vi "CalculateTorqueRipplevi.vi"(8 "error in (no error)":errorcluster, 11 "Torque Waveform":waveform(dbl)) -> (0 "error out":errorcluster, 3 "Torque Ripple (%)":dbl)   [LabVIEW 2017, in "McsaAnalysisFunctions.lvlib"]
uses:
  <vilib>/addons/InsightCM/Utilities/Analysis/MCSA/McsaAnalysisFunctions.lvlib
  <vilib>/Analysis/baseanly.llb/Mean (DBL).vi
  <vilib>/Waveform/WDTOps.llb/WDT Waveform Duration DBL.vi
  <vilib>/Waveform/WDTOps.llb/WDT Get Waveform Subset DBL.vi
  <vilib>/Analysis/NI_AALBase.lvlib
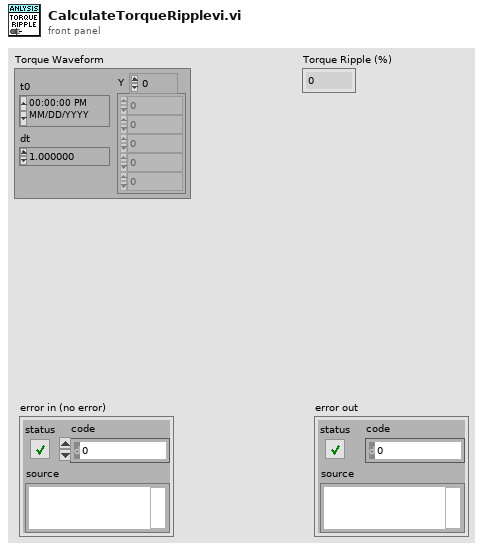
[diagram p1: front panel]
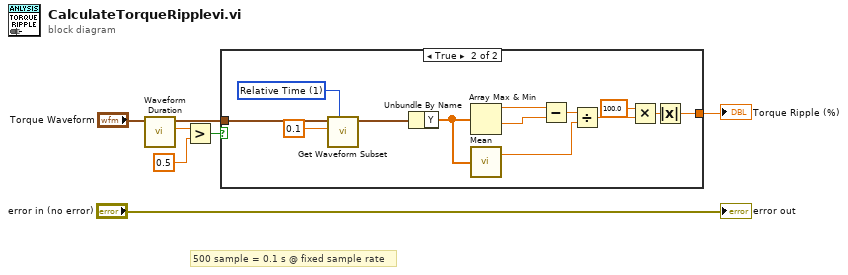
[diagram p0: block diagram]
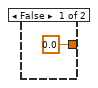
[diagram p2: hidden frame]
diagram:
  # "500 sample = 0.1 s @ fixed sample rate"
  n1 = call-poly <vilib>:"Waveform Duration.vi"("waveform in"="Torque Waveform") -> ("duration"=w5:dbl, "waveform out"=w6:waveform(dbl))  [unwired: 8 in, 1 out]
  n2 = Greater?(x=w5, y=0.5) -> (0:w2:bool)
  n3 = case shown="True" w2 {
    tunnel: w6 -> [_ w12]
    tunnel: [0.0 w11] -> w3
    frame False {
    }
    frame True {
      w10 = u16 1 items=["Samples", "Relative Time"] ("start/duration format")
      n4 = call-poly <vilib>:"Get Waveform Subset.vi"("start/duration format"=w10, "start samples/time"=0.1, "waveform in"=w12) -> ("waveform out"=w21:waveform(dbl))  [unwired: 3 in, 3 out]
      n5 = Unbundle By Name(w21) -> ("Y"=w20:dbl[])
      n6 = Array Max & Min(array=w20) -> (max value=w19:dbl, min value=w18:dbl)  [unwired: 2 out]
      n7 = call-poly <vilib>:"Mean.vi"("X"=w20) -> ("mean"=w16:dbl)  [unwired: 1 out]
      n8 = Subtract(x=w19, y=w18) -> (x-y=w17:dbl)
      n9 = Divide(x=w17, y=w16) -> (x/y=w15:dbl)
      n10 = Multiply(x=100.0, y=w15) -> (x*y=w13:dbl)
      n11 = Absolute Value(x=w13) -> (abs(x)=w11:dbl)
    }
  }
  "Torque Ripple (%)" <- w3
  "error out" <- "error in (no error)"
